vi "Generate Simulated Data.vi"(8 "error in (no error)":errorcluster, 10 "Display":refnum<queue>, 11 "Hardware Resources in":T1) -> (0 "error out":errorcluster)   [LabVIEW 2025, in "Acquisition.lvlib"]
doc: "Generates sample waveforms according to the signal type in the HW Config input."
uses:
  Acquisition.lvlib
  Acquistion_Configuration.ctl
  Signal Type.ctl
  support/Message Queue/Message Cluster.ctl
  controls/Get_Set_Enum.ctl
  controls/Pressure_Flow_Point.ctl
  controls/Mode Enum.ctl
  <userlib>/_OpenG.lib/numeric/numeric.llb/Random Number Within Range - DBL__ogtk.vi
  support/Message Queue/Enqueue Message (Single).vi
  controls/Calibration_Data.ctl
  <userlib>/_OpenG.lib/numeric/numeric.llb/openg_numeric__ogtk.lvlib
  support/Message Queue/Message Queue.lvlib
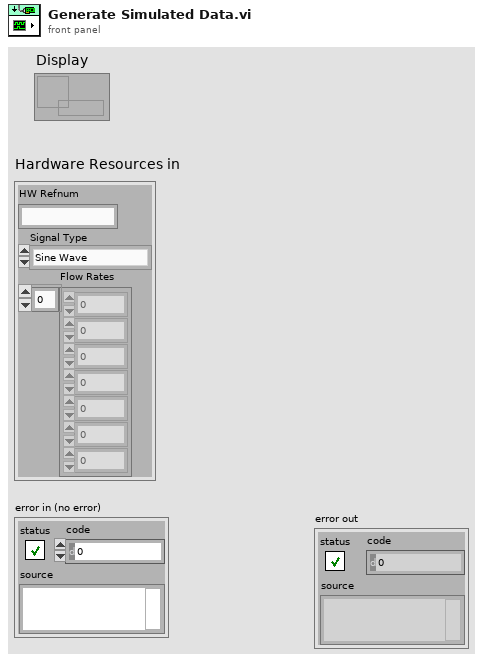
[diagram p1: front panel]
types:
  T1 = typedef "Acquisition.lvlib/Acquistion_Configuration.ctl" = cluster{"HW Refnum":string, "Signal Type":T2, "Flow Rates":dbl[]}
  T2 = typedef "Acquisition.lvlib/Signal Type.ctl" = enum16{"Sine Wave", "Square with Noise"}
  T3 = typedef "Pressure_Flow_Point.ctl" = cluster{"X (m_dot)":dbl[], "Y (sigma_delta_p)":dbl[]}
  T4 = cluster{"XY Graph":T3[], "Pass/Fail":cluster{"error_pct":dbl[], "pass_fail":dbl[]}}
  T5 = typedef "Get_Set_Enum.ctl" = enum16{"Get Design Tuners", "Set Design Tuners", "Get Design Constants", "Set Design Constants"}
  T6 = typedef "Mode Enum.ctl" = enum16{"Design", "Calibration"}
  T7 = typedef "Calibration_Data.ctl" = cluster{"Flow Rate (LBM/MIN)":dbl, "Pressure Ambient (PSIA)":dbl, "Pressure Inlet (PSIG)":dbl, "Pressure Tap (PSIG)":dbl, "Temperature Ambient (DEG F)":dbl, "Temperature Inlet (DEG F)":dbl, "Temperature Tap (DEG F)":dbl}
  T8 = typedef "Constants.ctl" = cluster{"P_amb (psia)":dbl, "T_in (Deg F)":dbl, "R_air (ft*lbf)/(lbm*R)":dbl, "g_c (lbm*ft)/(lbf*s^2)":dbl, "specific heat ratio":dbl, "Viscousity (lbm)/(ft*s)":dbl, "Cd":dbl, "Mass Flow (lbm/min) vs. Pressure Drop (inH2O) - Real Data":dbl[][]}
  T9 = typedef "Tuners.ctl" = cluster{"Inlet Diameter (in)":dbl, "Outlet Diameter (in)":dbl, "Length (in)":dbl, "Pipe_Diameter (in)":dbl, "D_h (in)":dbl, "OAR":dbl, "Run Optimizer":bool}
  T10 = cluster{"out_m_dot_empirical":dbl, "out_sigma_delta_p_empirical":dbl}
  T11 = cluster{"out_m_dot_sim":dbl, "sigma_delta_p_sim":dbl}
  T12 = cluster{"out_m_dot_sim":dbl, "sigma_delta_p_tap":dbl}
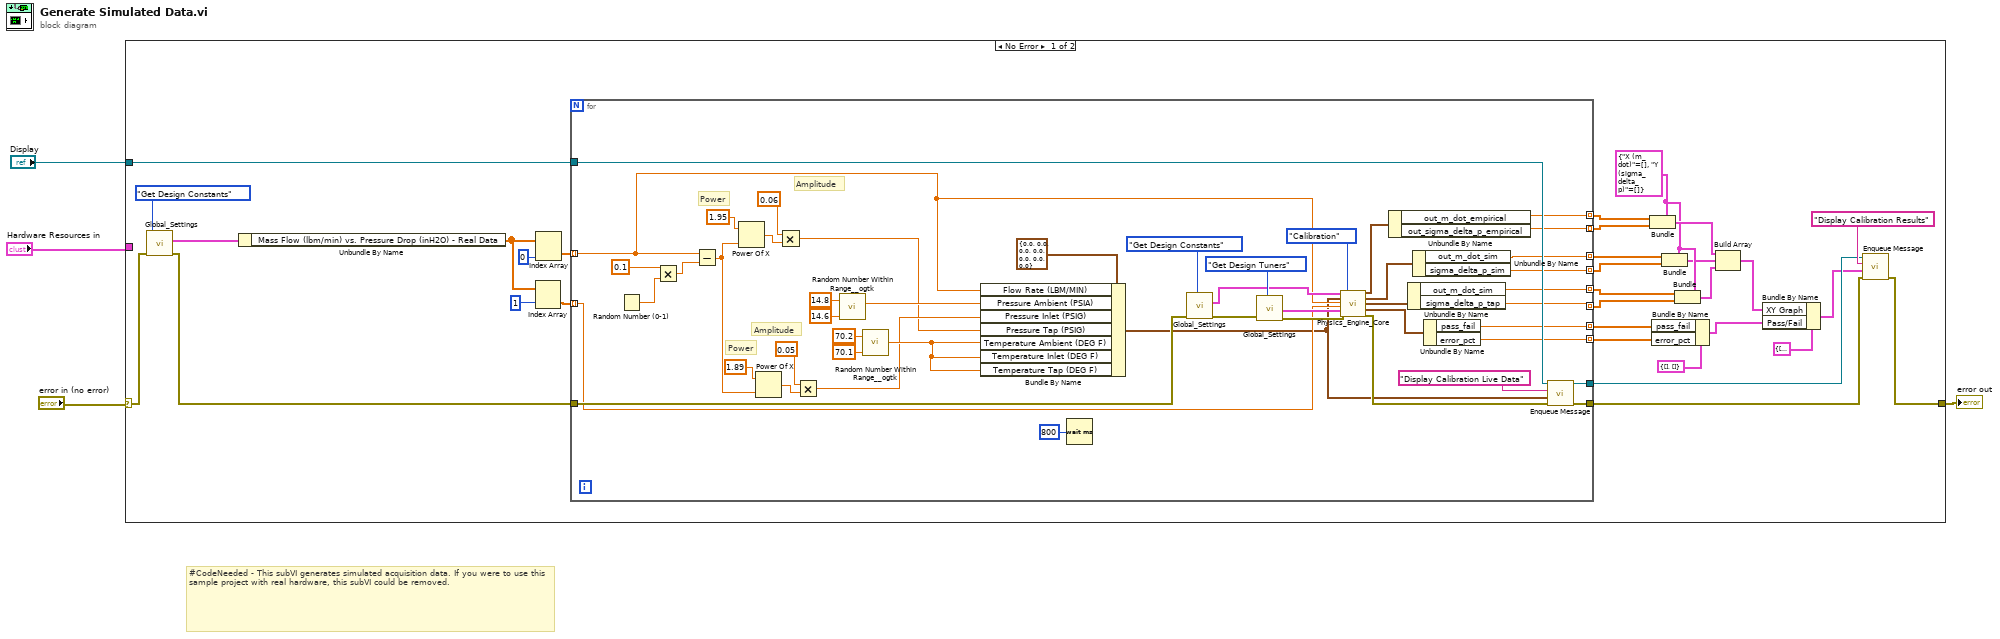
[diagram p0: block diagram]
diagram:
  # "#CodeNeeded - This subVI generates simulated acquisition data. If you were to use this sample project with real hardware, this subVI could be removed."
  n1 = case shown="No Error" "error in (no error)" {
    selector: "error in (no error)" -> [w30 w84]
    tunnel: [w17 w84] -> w1
    tunnel: "Hardware Resources in" -> [_ _]
    tunnel: "Display" -> [w35 _]
    frame No Error {
      w20 = T3 {"X (m_dot)"=[], "Y (sigma_delta_p)"=[]} ("XY_Plot_Data")
      n2 = call "Global_Settings.vi"("Enum"=Get_Set_Enum."Get Design Constants", "error in"=w30) -> ("error out"=w29:errorcluster, "Design Constants Out"=w33:T8)  [unwired: 7 in, 1 out]
      n3 = Unbundle By Name(w33) -> ("Mass Flow (lbm/min) vs. Pressure Drop (inH2O) - Real Data"=w13:dbl[][])
      n4 = Index Array(array=w13, index (col)=1 ("disabled index (col)")) -> (element=w12:dbl[])  [unwired: 1 in]
      n5 = Index Array(array=w13, index (col)=0 ("disabled index (col)")) -> (element=w31:dbl[])  [unwired: 1 in]
      n6 = for {
        tunnel: w29 -> [w53]
        tunnel: w35 -> [w62]
        tunnel: [w61] -> w15
        tunnel: [w60] -> w16
        tunnel: w31 -> [w40] mode=indexing
        tunnel: [w49] -> w28 mode=indexing
        tunnel: [w48] -> w27 mode=indexing
        tunnel: [w46] -> w22 mode=indexing
        tunnel: [w45] -> w21 mode=indexing
        tunnel: [w43] -> w24 mode=indexing
        tunnel: [w42] -> w23 mode=indexing
        tunnel: w12 -> [w41] mode=indexing
        tunnel: [w37] -> w10 mode=indexing
        tunnel: [w36] -> w9 mode=indexing
        # "Power"
        # "Amplitude"
        # "Power"
        # "Amplitude"
        n7 = Random Number (0-1)() -> (number: 0 to 1=w77:dbl)
        n8 = Multiply(x=0.1 ("High"), y=w77) -> (x*y=w76:dbl)
        n9 = Subtract(x=w40, y=w76) -> (x-y=w65:dbl)
        n10 = Power Of X(1:w65, 2:1.95 ("High")) -> (0:w73:dbl)
        n11 = Power Of X(1:w65, 2:1.89 ("High")) -> (0:w69:dbl)
        n12 = Multiply(x=0.06 ("High"), y=w73) -> (x*y=w64:dbl)
        n13 = Multiply(x=0.05 ("High"), y=w69) -> (x*y=w67:dbl)
        n14 = call-poly <userlib>:"Random Number Within Range__ogtk.vi"("High"=14.8, "Low"=14.6) -> ("Random Number"=w80:dbl)  [unwired: 3 in]
        n15 = call-poly <userlib>:"Random Number Within Range__ogtk.vi"("High"=70.2, "Low"=70.1) -> ("Random Number"=w71:dbl)  [unwired: 3 in]
        n16 = Bundle By Name(cluster=T7 {"Flow Rate (LBM/MIN)"=0.0, "Pressure Ambient (PSIA)"=0.0, "Pressure Inlet (PSIG)"=0.0, "Pressure Tap (PSIG)"=0.0, "Temperature Ambient (DEG F)"=0.0, "Temperature Inlet (DEG F)"=0.0, "Temperature Tap (DEG F)"=0.0} ("Calibration Data 2"), "Flow Rate (LBM/MIN)"=w40, "Pressure Ambient (PSIA)"=w80, "Pressure Inlet (PSIG)"=w67, "Pressure Tap (PSIG)"=w64, "Temperature Ambient (DEG F)"=w71, "Temperature Inlet (DEG F)"=w71, "Temperature Tap (DEG F)"=w71) -> (w39:T7)
        n17 = Wait (ms)(milliseconds to wait=u32 800) -> ()  [unwired: 1 out]
        n18 = call "Global_Settings.vi"("Enum"=Get_Set_Enum."Get Design Constants", "error in"=w53) -> ("error out"=w54:errorcluster, "Design Constants Out"=w51:T8)  [unwired: 7 in, 1 out]
        n19 = call "Global_Settings.vi"("Enum"=Get_Set_Enum."Get Design Tuners", "error in"=w54) -> ("error out"=w58:errorcluster, "Design Tuners Out"=w52:T9)  [unwired: 7 in, 1 out]
        n20 = call "Physics_Engine_Core.vi"("Design Constants"=w51, "Calibration Data"=w39, "m_dot_empirical"=w40, "sigma_delta_p_empirical"=w41, "Design Tuners"=w52, "error in (no error)"=w58, "Enum"=Mode_Enum."Calibration") -> ("empirical curve"=w50:T10, "sim curve"=w47:T11, "tap curve"=w44:T12, "success/failure"=w38:cluster{"pass_fail":dbl, "error_pct":dbl}, "error out"=w57:errorcluster)  [unwired: 7 in, 1 out]
        n21 = Unbundle By Name(w50) -> ("out_m_dot_empirical"=w49:dbl, "out_sigma_delta_p_empirical"=w48:dbl)
        n22 = Unbundle By Name(w44) -> ("out_m_dot_sim"=w43:dbl, "sigma_delta_p_tap"=w42:dbl)
        n23 = Unbundle By Name(w47) -> ("out_m_dot_sim"=w46:dbl, "sigma_delta_p_sim"=w45:dbl)
        n24 = Unbundle By Name(w38) -> ("pass_fail"=w37:dbl, "error_pct"=w36:dbl)
        n25 = call-poly "Enqueue Message.vi"("error in (no error)"=w57, "Message Data"=w39, "Message"="Display Calibration Live Data", "Message Queue"=w62) -> ("error out"=w61:errorcluster, "dup Message Queue"=w60:refnum<queue>)  [unwired: 6 in]
      }
      n26 = Bundle(cluster=w20, "X (m_dot)"=w28, "Y (sigma_delta_p)"=w27) -> (w26:T3)
      n27 = Bundle By Name(cluster=cluster{"error_pct":dbl[], "pass_fail":dbl[]} {"error_pct"=[], "pass_fail"=[]}, "pass_fail"=w10, "error_pct"=w9) -> (w5:cluster{"error_pct":dbl[], "pass_fail":dbl[]})
      n28 = Bundle(cluster=w20, "X (m_dot)"=w22, "Y (sigma_delta_p)"=w21) -> (w19:T3)
      n29 = Bundle(cluster=w20, "X (m_dot)"=w24, "Y (sigma_delta_p)"=w23) -> (w18:T3)
      n30 = Build Array(w26, w19, w18) -> (w8:T3[])
      n31 = Bundle By Name(cluster=T4 {"XY Graph"=[], "Pass/Fail"={"error_pct"=[], "pass_fail"=[]}}, "XY Graph"=w8, "Pass/Fail"=w5) -> (w7:T4)
      n32 = call-poly "Enqueue Message.vi"("error in (no error)"=w15, "Message Data"=w7, "Message"="Display Calibration Results", "Message Queue"=w16) -> ("error out"=w17:errorcluster)  [unwired: 6 in, 1 out]
    }
    frame Error {
    }
  }
  "error out" <- w1
